vi "Binary Confusion Matrix.vi"(9 "True Label":i32=1 caption="True Label (1)", 10 "Actual Labels":dbl[](array[numeric]), 11 "Predicted Labels":dbl[](array[numeric])) -> (3 "Binary Confusion Matrix":T1)   [LabVIEW 2014]
uses:
  Controls/Binary_ConfusionMatrix.ctl
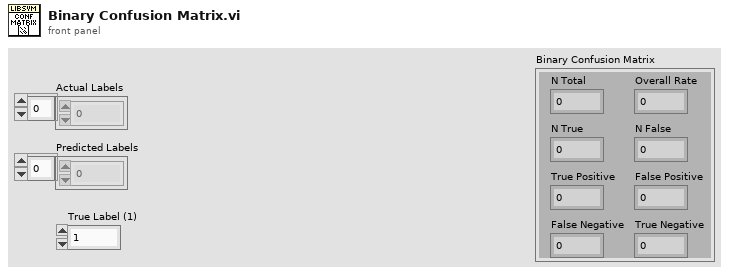
[diagram p1: front panel]
types:
  T1 = typedef "Binary_ConfusionMatrix.ctl" = cluster{"N Total":u32, "N True":u32, "N False":u32, "Overall Rate":dbl, "True Positive":dbl, "False Positive":dbl, "False Negative":dbl, "True Negative":dbl}
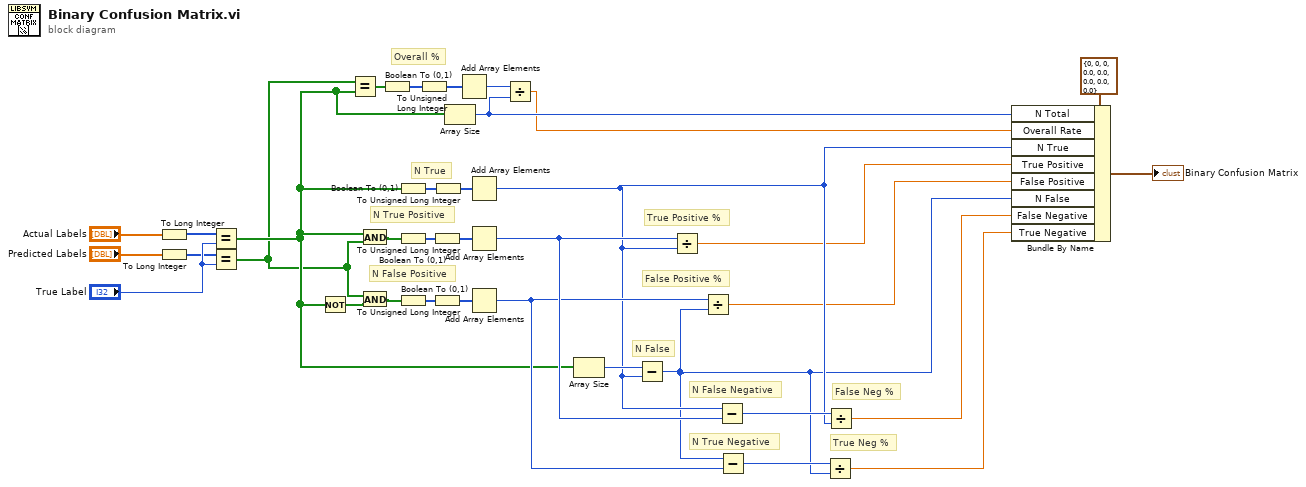
[diagram p0: block diagram]
diagram:
  # "True Neg %"
  # "False Neg %"
  # "False Positive %"
  # "True Positive %"
  # "Overall %"
  # "N False Negative"
  # "N True Negative"
  # "N False"
  # "N False Positive"
  # "N True Positive"
  # "N True"
  n1 = To Long Integer(number="Actual Labels") -> (32bit integer=w12:i32[])
  n2 = To Long Integer(number="Predicted Labels") -> (32bit integer=w11:i32[])
  n3 = Equal?(x=w12, y="True Label") -> (x = y?=w10:bool[])
  n4 = Equal?(x=w11, y="True Label") -> (x = y?=w9:bool[])
  n5 = Not(x=w10) -> (.not. x?=w23:bool[])
  n6 = Equal?(x=w9, y=w10) -> (x = y?=w20:bool[])
  n7 = And(x=w10, y=w9) -> (x .and. y?=w29:bool[])
  n8 = And(x=w9, y=w23) -> (x .and. y?=w24:bool[])
  n9 = Boolean To (0,1)(Boolean=w20) -> (0, 1=w21:i16[])
  n10 = Boolean To (0,1)(Boolean=w10) -> (0, 1=w31:i16[])
  n11 = Boolean To (0,1)(Boolean=w29) -> (0, 1=w28:i16[])
  n12 = Boolean To (0,1)(Boolean=w24) -> (0, 1=w25:i16[])
  n13 = To Unsigned Long Integer(number=w21) -> (unsigned 32bit integer=w19:u32[])
  n14 = To Unsigned Long Integer(number=w28) -> (unsigned 32bit integer=w27:u32[])
  n15 = To Unsigned Long Integer(number=w25) -> (unsigned 32bit integer=w26:u32[])
  n16 = To Unsigned Long Integer(number=w31) -> (unsigned 32bit integer=w30:u32[])
  n17 = Array Size(array=w10) -> (size(s)=w8:i32)
  n18 = Add Array Elements(numeric array=w19) -> (sum=w14:u32)
  n19 = Add Array Elements(numeric array=w30) -> (sum=w6:u32)
  n20 = Add Array Elements(numeric array=w27) -> (sum=w18:u32)
  n21 = Add Array Elements(numeric array=w26) -> (sum=w17:u32)
  n22 = Divide(x=w14, y=w8) -> (x/y=w7:dbl)
  n23 = Array Size(array=w10) -> (size(s)=w22:i32)
  n24 = Subtract(x=w22, y=w6) -> (x-y=w1:u32)
  n25 = Divide(x=w18, y=w6) -> (x/y=w5:dbl)
  n26 = Divide(x=w17, y=w1) -> (x/y=w4:dbl)
  n27 = Subtract(x=w6, y=w18) -> (x-y=w16:u32)
  n28 = Subtract(x=w1, y=w17) -> (x-y=w15:u32)
  n29 = Divide(x=w15, y=w1) -> (x/y=w2:dbl)
  n30 = Divide(x=w16, y=w6) -> (x/y=w3:dbl)
  n31 = Bundle By Name(cluster=T1 {"N Total"=0, "N True"=0, "N False"=0, "Overall Rate"=0.0, "True Positive"=0.0, "False Positive"=0.0, "False Negative"=0.0, "True Negative"=0.0} ("Binary Confusion Matrix"), "N Total"=w8, "Overall Rate"=w7, "N True"=w6, "True Positive"=w5, "False Positive"=w4, "N False"=w1, "False Negative"=w3, "True Negative"=w2) -> (→"Binary Confusion Matrix":T1)
